vi "HFR500 Create String.vi"(3 "Ch number":i32=1 min=0 max=4, 4 "Command":string, 5 "ppm Range":T1) -> (1 "TX String (ASCII)":string, 2 "TX String (hex)":string)   [LabVIEW 2020]
uses:
  HFR500 ppm Range.ctl
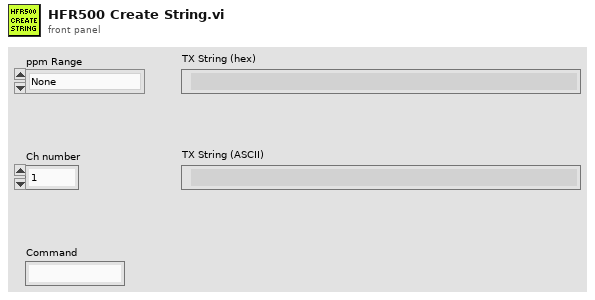
[diagram p1: front panel]
types:
  T1 = typedef "HFR500 ppm Range.ctl" = enum16{"None", "1,000", "2,000", "5,000", "10,000", "20,000", "50,000", "100,000", "200,000"}
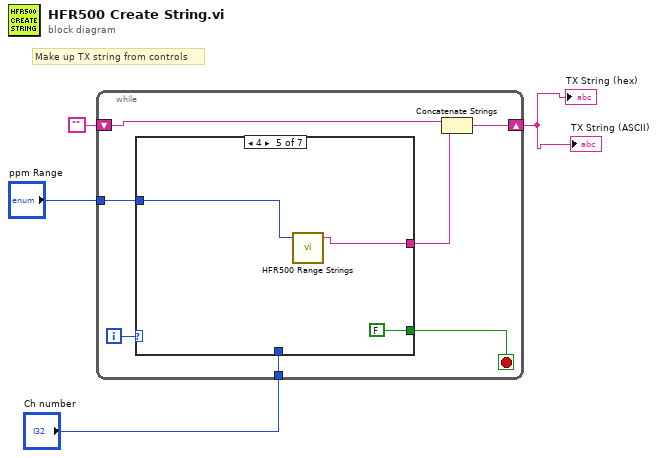
[diagram p0: block diagram]
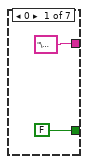
[diagram p2: hidden frame]
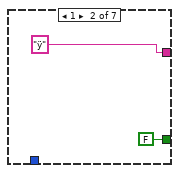
[diagram p3: hidden frame]
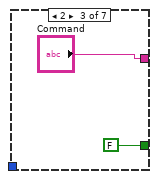
[diagram p4: hidden frame]
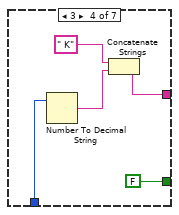
[diagram p5: hidden frame]
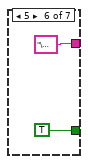
[diagram p6: hidden frame]
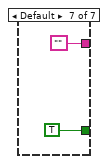
[diagram p7: hidden frame]
diagram:
  # "Make up TX string from controls"
  n1 = while {
    shift-right: [w9] -> w1
    shift-left: "" -> [w8]
    tunnel: "Ch number" -> [w6]
    tunnel: "ppm Range" -> [w5]
    i -> [w11]
    stop <- w10 stop-if-true
    n2 = case shown="4" w11 {
      tunnel: [FALSE FALSE FALSE FALSE FALSE TRUE TRUE] -> w10
      tunnel: ["\u0002" "ÿ" ("Don't Care Byte") "Command" w21 w24 "\u0003" ""] -> w7
      tunnel: w6 -> [_ _ _ w18 _ _ _]
      tunnel: w5 -> [_ _ _ _ w23 _ _]
      frame 0 {
      }
      frame 1 {
      }
      frame 2 {
      }
      frame 3 {
        n3 = Number To Decimal String(number=w18) -> (decimal integer string=w19:string)  [unwired: 1 in]
        n4 = Concatenate Strings(" K", w19) -> (w21:string)
      }
      frame 4 {
        n5 = call "HFR500 Range Strings.vi"("ppm Range"=w23) -> ("Range String"=w24:string)  [unwired: 3 in, 1 out]
      }
      frame 5 {
      }
      frame Default {
      }
    }
    n6 = Concatenate Strings(w8, w7) -> (w9:string)
  }
  "TX String (hex)" <- w1
  "TX String (ASCII)" <- w1
